vi "Lab4_2.vi"() -> ()   [LabVIEW 2021]
uses:
  <vilib>/Simulation/DataSources/Implementation/NILVSim Signal Generator.llb/SIM Signal Generator (scalar).vi
  <vilib>/Simulation/Implementation/XNodeFramework/SimXNode/SimX.xnode
  <vilib>/Simulation/SignalDisplay/Implementation/NILVSim Time Waveform.llb/SIM Time Waveform (vector).vi
  <vilib>/Simulation/ContinuousLinear/Implementation/NILVSim Transfer Function.llb/SIM Transfer Function (SISO).vi
  <vilib>/Simulation/SignalArithmetic/Implementation/NILVSim Gain.llb/SIM Gain (scalar).vi
  <vilib>/Simulation/ContinuousLinear/Implementation/NILVSim Integrator new.llb/SIM Integrator (scalar).vi
  <vilib>/Simulation/ContinuousLinear/Implementation/NILVSim Transfer Function Direct.llb/SIM Transfer Function Direct (SISO).vi
  <vilib>/Simulation/Implementation/Shared/SIMSCR Execution Mode.ctl
  <vilib>/Simulation/Scripting/Companion Diagram/SimConfigNode/_simSolvers.ctl
  <vilib>/Simulation/Scripting/Companion Diagram/SimConfigNode/SimParams.ctl
  <vilib>/Simulation/Scripting/Companion Diagram/SimConfigNode/SimDog.xnode
panel:
  out "Waveform Chart":waveform(dbl)[](graph)
  in  "Kp 2":dbl
  in  "Ki 2":dbl
  in  "Kd 2":dbl
  in  "Vpos":dbl
  in  "Cpos":dbl
  in  "Vneg":dbl
  in  "Cneg":dbl
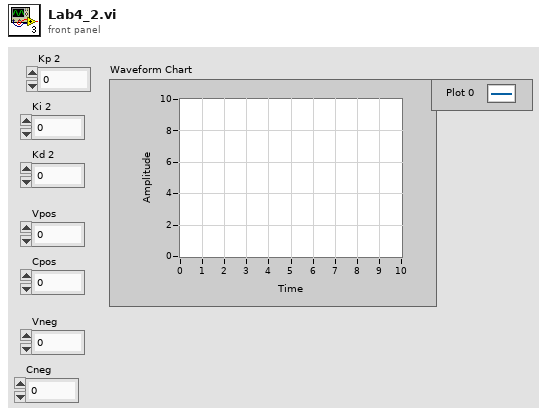
[diagram p1: front panel]
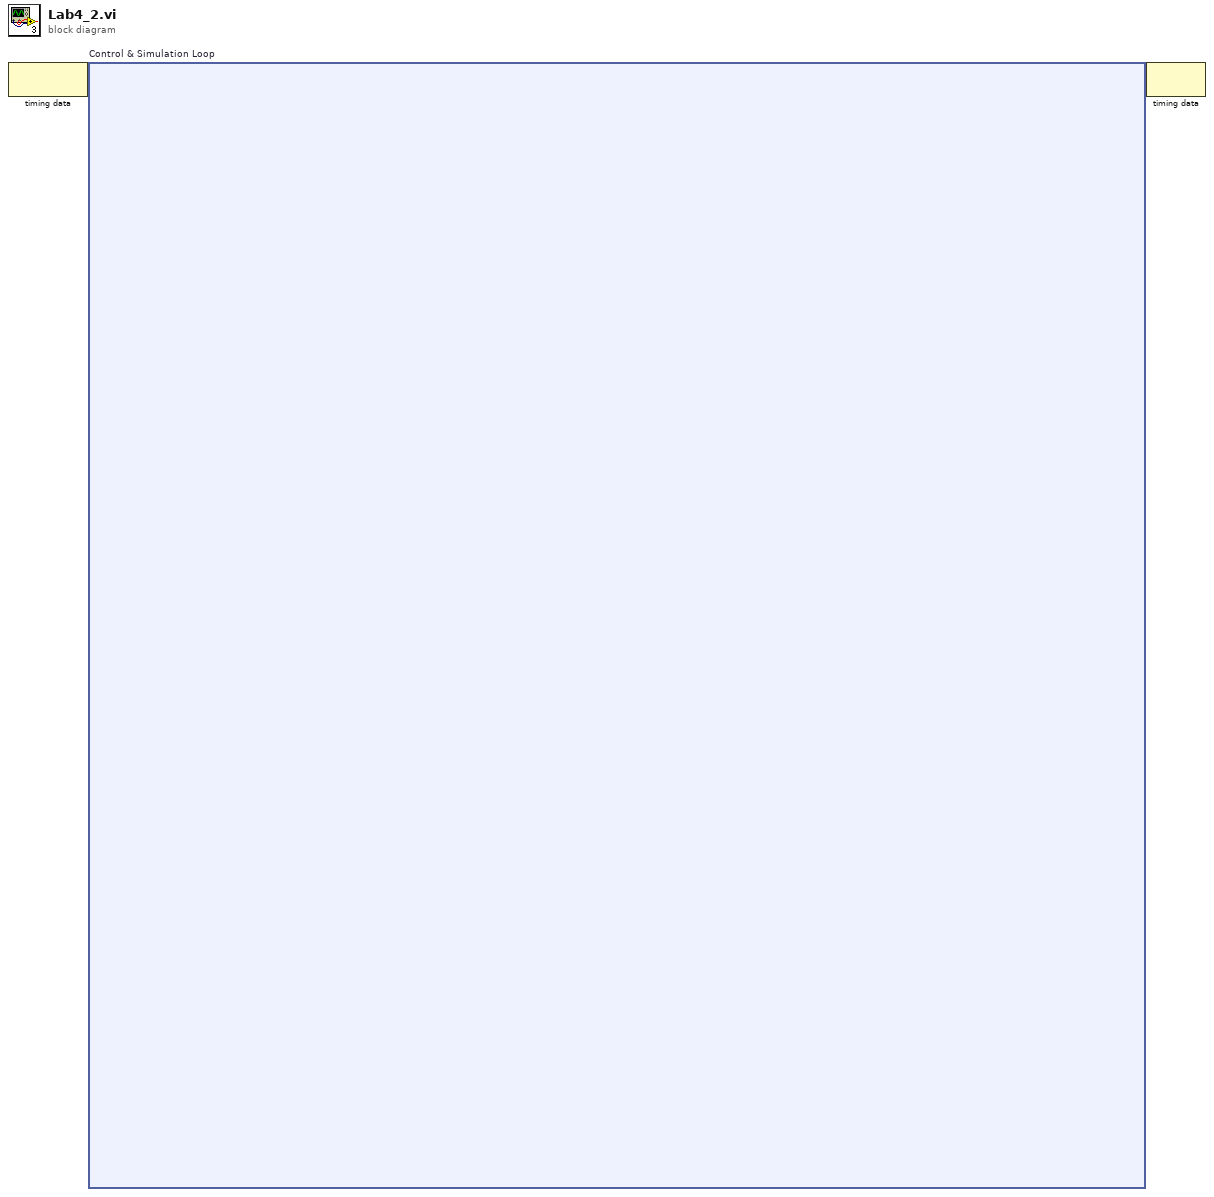
[diagram p0: block diagram]
diagram:
  n1 = node-c288() -> (w2:variant)  [unwired: 1 in]
  n2 = node-c254 "Control & Simulation Loop"(w2) -> (w1:variant)
  n3 = node-c288(w1) -> ()  [unwired: 1 out]
